vi "GenerateFarfiledGrid.vi"(3 "thetaPicth":dbl, 4 "thetaRol":dbl, 5 "L":dbl) -> (0 "PitchGrid":dbl[](array[numeric]), 1 "RollGrid":dbl[](array[numeric]))   [LabVIEW 2018]
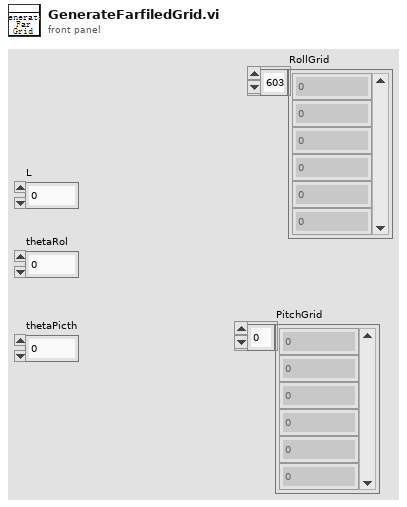
[diagram p1: front panel]
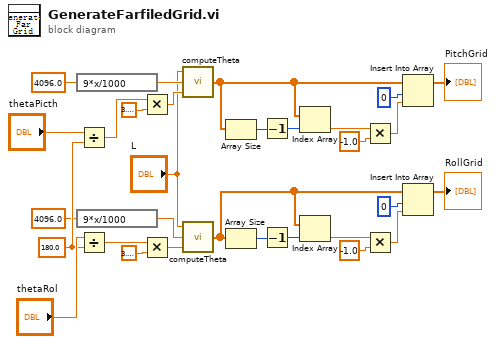
[diagram p0: block diagram]
diagram:
  w25 = 180.0 ("y")
  n1 = expression code="9*x/1000"(4096.0) -> (w18:dbl)
  n2 = expression code="9*x/1000"(4096.0) -> (w19:dbl)
  n3 = Divide(x="thetaPicth", y=w25) -> (x/y=w24:dbl)
  n4 = Divide(x="thetaRol", y=w25) -> (x/y=w30:dbl)
  n5 = Multiply(x=w24, y=3.141592653589793) -> (x*y=w22:dbl)
  n6 = Multiply(x=w30, y=3.141592653589793) -> (x*y=w27:dbl)
  n7 = call "computeTheta.vi"("thetaT"=w22, "M"=w18, "L"="L") -> ("ThetaOut"=w1:dbl[])  [unwired: 2 in]
  n8 = call "computeTheta.vi"("thetaT"=w27, "M"=w19, "L"="L") -> ("ThetaOut"=w15:dbl[])  [unwired: 2 in]
  n9 = Array Size(array=w1) -> (size(s)=w7:i32)
  n10 = Array Size(array=w15) -> (size(s)=w14:i32)
  n11 = Decrement(x=w7) -> (x-1=w6:i32)
  n12 = Decrement(x=w14) -> (x-1=w13:i32)
  n13 = Index Array(array=w1, index=w6) -> (element=w5:dbl)
  n14 = Index Array(array=w15, index=w13) -> (element=w12:dbl)
  n15 = Multiply(x=w5, y=-1.0) -> (x*y=w3:dbl)
  n16 = Multiply(x=w12, y=-1.0) -> (x*y=w10:dbl)
  n17 = Insert Into Array(array=w1, index=0, new element=w3) -> (→"PitchGrid":dbl[])
  n18 = Insert Into Array(array=w15, index=0, new element=w10) -> (→"RollGrid":dbl[])
